vi "Set Exposure Time.vi"(8 "error in (no error)":errorcluster, 11 "CCDCamera in":refnum<class "CCDCamera.lvclass">) -> (0 "error out":errorcluster, 3 "CCDCamera out":refnum<class "CCDCamera.lvclass">)   [LabVIEW 2018, in "CCDCamera.lvclass"]
uses:
  CCDCamera.lvclass
  C:/Users/observer/Desktop/SPARC4_ACS/SPARC4_ACS/Simulated_CCD_Camera/Simulated_CCD_Camera.lvclass
  Simulated_CCD_Camera/Simulated_CCD_Camera.lvclass/Simulated_CCD_Camera.ctl
  Interface/Interface.lvclass/Interface.ctl
  Interface/Interface.lvclass
  Simulated_CCD_Camera/Simulated_CCD_Camera.lvclass
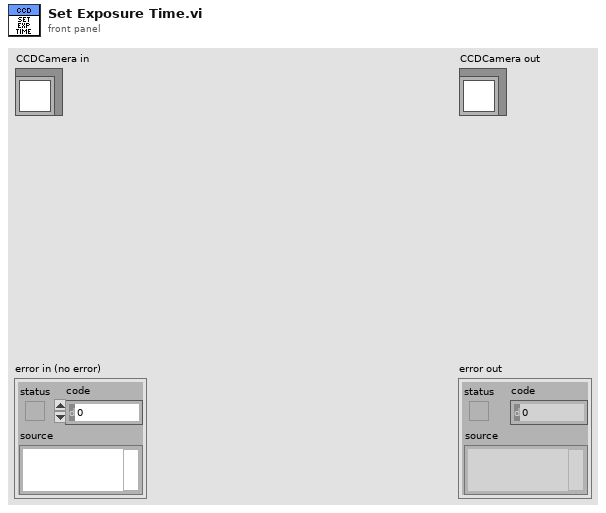
[diagram p1: front panel]
types:
  T1 = cluster{"COOLER_POWER_STATUS":u16, "TEMP":i32, "EXPTIME":dbl, "#FRAMES":u32, "#CUBES":u32}
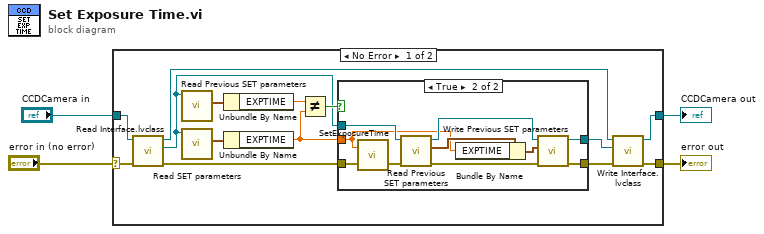
[diagram p0: block diagram]
diagram:
  n1 = case shown="No Error" "error in (no error)" {
    selector: "error in (no error)" -> [w18 w32]
    tunnel: [w15 w32] -> w2
    tunnel: [w14 w31] -> w1
    tunnel: "CCDCamera in" -> [w13 w31]
    frame No Error {
      n2 = call "Read Interface.lvclass.vi"("error in (no error)"=w18, "Simulated_CCD_Camera in"=w13) -> ("error out"=w10:errorcluster, "Interface.lvclass"=w5:refnum<class "Interface.lvclass">, "Simulated_CCD_Camera out"=w16:refnum<class "CCDCamera.lvclass">)  [unwired: 7 in]
      n3 = call "Read Previous SET parameters.vi"("Interface in"=w5) -> ("Previous SET parameters"=w8:T1)  [unwired: 8 in, 2 out]
      n4 = call "Read SET parameters.vi"("Interface in"=w5) -> ("SET parameters"=w9:T1)  [unwired: 8 in, 2 out]
      n5 = Unbundle By Name(w8) -> ("EXPTIME"=w7:dbl)
      n6 = Unbundle By Name(w9) -> ("EXPTIME"=w6:dbl)
      n7 = Not Equal?(x=w7, y=w6) -> (x != y?=w17:bool)
      n8 = case shown="True" w17 {
        tunnel: w6 -> [_ w21]
        tunnel: w5 -> [w20 w29]
        tunnel: [w20 w23] -> w12
        tunnel: [w19 w24] -> w11
        tunnel: w10 -> [w19 w30]
        frame False {
        }
        frame True {
          n9 = call <userlib>:"SetExposureTime.vi"("error in (no error)"=w30, "time"=w21) -> ("error out"=w28:errorcluster)  [unwired: 1 out]
          n10 = call "Read Previous SET parameters.vi"("error in (no error)"=w28, "Interface in"=w29) -> ("error out"=w22:errorcluster, "Previous SET parameters"=w27:T1, "Interface out"=w25:refnum<class "Interface.lvclass">)  [unwired: 7 in]
          n11 = Bundle By Name(cluster=w27, "EXPTIME"=w21) -> (w26:T1)
          n12 = call "Write Previous SET parameters.vi"("error in (no error)"=w22, "Previous SET parameters"=w26, "Interface in"=w25) -> ("error out"=w24:errorcluster, "Interface out"=w23:refnum<class "Interface.lvclass">)  [unwired: 7 in]
        }
      }
      n13 = call "Write Interface.lvclass.vi"("error in (no error)"=w11, "Interface.lvclass"=w12, "Simulated_CCD_Camera in"=w16) -> ("error out"=w15:errorcluster, "Simulated_CCD_Camera out"=w14:refnum<class "CCDCamera.lvclass">)  [unwired: 7 in]
    }
    frame Error {
    }
  }
  "error out" <- w2
  "CCDCamera out" <- w1
